vi "_Adjust Dynamic_simple.vi"(8 "error in (no error)":errorcluster, 10 "Image Dst":T1, 11 "Image Src":T1) -> (0 "error out":errorcluster, 3 "Image Out":T1)   [LabVIEW 2015]
doc: "Redistributes the pixel values of an image in order to use the full dynamic range of the image."
uses:
  <vilib>/vision/NI_Vision_Development_Module.lvlib
  <vilib>/vision/Image Controls.llb/IMAQ Image.ctl
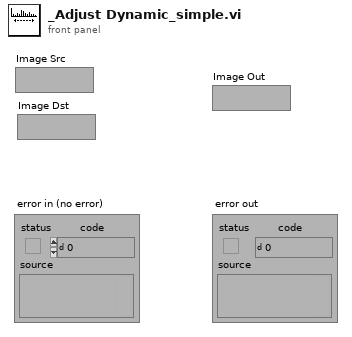
[diagram p1: front panel]
types:
  T1 = typedef "IMAQ Image.ctl" = refnum<image>
  T2 = typedef "Image Type" = u32
  T3 = cluster{"histogram":u32[], "Minimal Value":sgl, "Maximal Value":sgl, "Starting Value":sgl, "Interval Width":sgl, "Mean Value":sgl, "Standard  Variation":sgl, "Area (pixels)":i32}
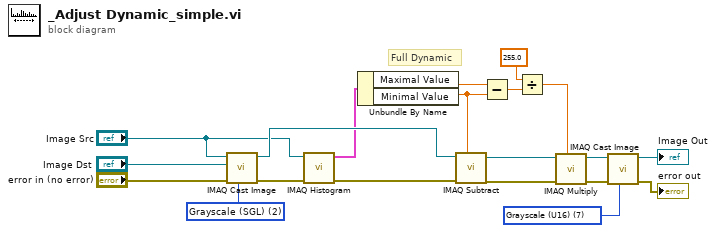
[diagram p0: block diagram]
diagram:
  w1 = T2 7 items=["Grayscale (U8)", "Grayscale (I16)", "Grayscale (SGL)", "Complex (CSG)", "RGB (U32)", "HSL (U32)", "RGB (U64)", "Grayscale (U16)"] ("Image Type")
  w5 = T2 2 items=["Grayscale (U8)", "Grayscale (I16)", "Grayscale (SGL)", "Complex (CSG)", "RGB (U32)", "HSL (U32)", "RGB (U64)"] ("Image Type")
  # "Full Dynamic"
  n1 = call "IMAQ Cast Image"("Image Type"=w5, "error in (no error)"="error in (no error)", "Image Dst"="Image Dst", "Image Src"="Image Src") -> ("error out"=w8:errorcluster, "Image Dst Out"=w17:T1)  [unwired: 6 in]
  n2 = call "IMAQ Histogram"("error in (no error)"=w8, "Image"="Image Src") -> ("error out"=w7:errorcluster, "Histogram Report"=w4:T3)  [unwired: 8 in]
  n3 = Unbundle By Name(w4) -> ("Maximal Value"=w3:sgl, "Minimal Value"=w2:sgl)
  n4 = call "IMAQ Subtract"("Image Src A"=w17, "Constant"=w2, "error in (no error)"=w7) -> ("Image Dst Out"=w18:T1, "error out"=w15:errorcluster)  [unwired: 4 in]
  n5 = Subtract(x=w3, y=w2) -> (x-y=w19:sgl)
  n6 = Divide(x=sgl 255.0 ("8 bit"), y=w19) -> (x/y=w16:sgl)
  n7 = call "IMAQ Multiply"("Image Src A"=w18, "Constant"=w16, "error in (no error)"=w15) -> ("Image Dst Out"=w14:T1, "error out"=w13:errorcluster)  [unwired: 4 in]
  n8 = call "IMAQ Cast Image"("Image Type"=w1, "error in (no error)"=w13, "Image Src"=w14) -> ("error out"=→"error out":errorcluster, "Image Dst Out"=→"Image Out":T1)  [unwired: 7 in]
